vi "Configuration - SWITCH Properties FGV.vi"(8 "error in (no error)":errorcluster, 11 "Parent Ref in":T1 format="%.0x") -> (0 "error out":errorcluster, 3 "Parent Ref out":T1 format="%.0x")   [LabVIEW 2015, in "DMM-SWITCH-ScanList System Explorer.lvlib"]
uses:
  DMM-SWITCH-ScanList System Explorer.lvlib
  <vilib>/NI Veristand/Custom Device API/Custom Device Item Ref.ctl
  <vilib>/NI Veristand/Custom Device API/Custom Device Channel.ctl
  <vilib>/NI Veristand/Custom Device API/Custom Device Channel Type.ctl
  Shared/Constants.vi
  <vilib>/NI Veristand/Custom Device API/Set Item Property (String).vi
  <vilib>/NI Veristand/Custom Device API/Set Item Property (Boolean).vi
  <vilib>/NI Veristand/Custom Device API/Set Item Property (String Array).vi
  <vilib>/NI Veristand/Custom Device API/Custom Device API.lvlib
  Shared/DMM-SWITCH-ScanList Shared.lvlib
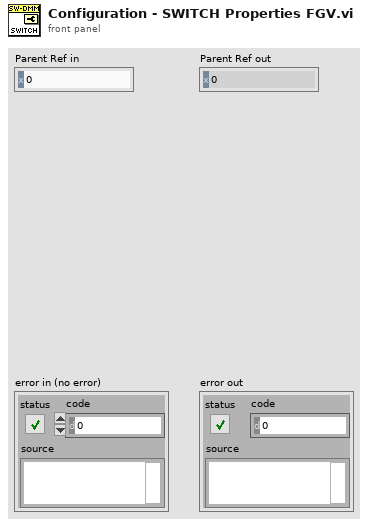
[diagram p1: front panel]
types:
  T1 = typedef "Custom Device API.lvlib/Custom Device Item Ref.ctl" = u64
  T2 = typedef "Custom Device API.lvlib/Custom Device Channel.ctl" = cluster{"Type":T3, "Units":string, "Default Value":dbl, "Faultable":bool, "Scalable":bool}
  T3 = typedef "Custom Device API.lvlib/Custom Device Channel Type.ctl" = enum16{"Input", "Output"}
  T4 = typedef "niSwitch Topologies.ctl" = string
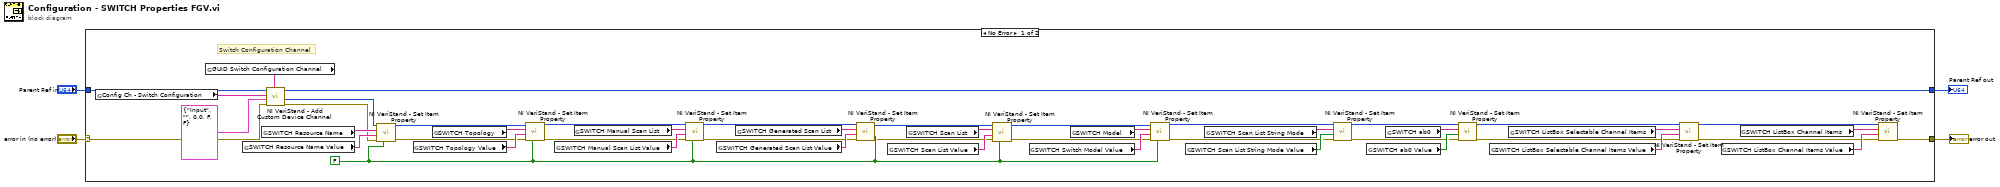
[diagram p0: block diagram]
diagram:
  n1 = case shown="No Error" "error in (no error)" {
    selector: "error in (no error)" -> [w6 w54]
    tunnel: [w18 w54] -> w4
    tunnel: [w9 w53] -> w3
    tunnel: "Parent Ref in" -> [w8 w53]
    frame No Error {
      w30 = FALSE ("Binary String (T)")
      # "Switch Configuration Channel"
      n2 = global read "Constants.vi" "Config Ch - Switch Configuration"() -> (w5:string)
      n3 = global read "Constants.vi" "GUID Switch Configuration Channel"() -> (w40:string)
      n4 = global read "Constants.vi" "SWITCH Resource Name Value"() -> (w31:string)
      n5 = global read "Constants.vi" "SWITCH Resource Name"() -> (w41:string)
      n6 = call <vilib>:"NI VeriStand - Add Custom Device Channel.vi"("GUID (Default Channel)"=w40, "error in (no error)"=w6, "Channel"=T2 {"Type"=enum."Input", "Units"="", "Default Value"=0.0, "Faultable"=FALSE, "Scalable"=FALSE}, "Channel Name"=w5, "Parent Ref in"=w8) -> ("error out"=w13:errorcluster, "Channel Ref"=w12:T1, "Parent Ref out"=w9:T1)  [unwired: 3 in, 1 out]
      n7 = call-poly <vilib>:"NI VeriStand - Set Item Property.vi"("Binary String (T)"=w30, "error in (no error)"=w13, "Value"=w31, "Property Name"=w41, "Item Ref in"=w12) -> ("error out"=w10:errorcluster, "Item Ref out"=w11:T1)  [unwired: 4 in, 1 out]
      n8 = global read "Constants.vi" "SWITCH Topology Value"() -> (w32:T4)
      n9 = global read "Constants.vi" "SWITCH Topology"() -> (w42:string)
      n10 = call-poly <vilib>:"NI VeriStand - Set Item Property.vi"("Binary String (T)"=w30, "error in (no error)"=w10, "Value"=w32, "Property Name"=w42, "Item Ref in"=w11) -> ("error out"=w15:errorcluster, "Item Ref out"=w14:T1)  [unwired: 4 in, 1 out]
      n11 = global read "Constants.vi" "SWITCH Manual Scan List Value"() -> (w33:string)
      n12 = global read "Constants.vi" "SWITCH Manual Scan List"() -> (w43:string)
      n13 = call-poly <vilib>:"NI VeriStand - Set Item Property.vi"("Binary String (T)"=w30, "error in (no error)"=w15, "Value"=w33, "Property Name"=w43, "Item Ref in"=w14) -> ("error out"=w24:errorcluster, "Item Ref out"=w25:T1)  [unwired: 4 in, 1 out]
      n14 = global read "Constants.vi" "SWITCH Generated Scan List Value"() -> (w44:string)
      n15 = global read "Constants.vi" "SWITCH Generated Scan List"() -> (w45:string)
      n16 = call-poly <vilib>:"NI VeriStand - Set Item Property.vi"("Binary String (T)"=w30, "error in (no error)"=w24, "Value"=w44, "Property Name"=w45, "Item Ref in"=w25) -> ("error out"=w28:errorcluster, "Item Ref out"=w26:T1)  [unwired: 4 in, 1 out]
      n17 = global read "Constants.vi" "SWITCH Scan List Value"() -> (w47:string)
      n18 = global read "Constants.vi" "SWITCH Scan List"() -> (w46:string)
      n19 = call-poly <vilib>:"NI VeriStand - Set Item Property.vi"("Binary String (T)"=w30, "error in (no error)"=w28, "Value"=w47, "Property Name"=w46, "Item Ref in"=w26) -> ("error out"=w29:errorcluster, "Item Ref out"=w27:T1)  [unwired: 4 in, 1 out]
      n20 = global read "Constants.vi" "SWITCH Switch Model Value"() -> (w34:string)
      n21 = global read "Constants.vi" "SWITCH Model"() -> (w48:string)
      n22 = call-poly <vilib>:"NI VeriStand - Set Item Property.vi"("Binary String (T)"=w30, "error in (no error)"=w29, "Value"=w34, "Property Name"=w48, "Item Ref in"=w27) -> ("error out"=w20:errorcluster, "Item Ref out"=w19:T1)  [unwired: 4 in, 1 out]
      n23 = global read "Constants.vi" "SWITCH Scan List String Mode Value"() -> (w35:bool)
      n24 = global read "Constants.vi" "SWITCH Scan List String Mode"() -> (w49:string)
      n25 = call-poly <vilib>:"NI VeriStand - Set Item Property.vi"("error in (no error)"=w20, "Value"=w35, "Property Name"=w49, "Item Ref in"=w19) -> ("error out"=w21:errorcluster, "Item Ref out"=w22:T1)  [unwired: 5 in, 1 out]
      n26 = global read "Constants.vi" "SWITCH ab0 Value"() -> (w36:bool)
      n27 = global read "Constants.vi" "SWITCH ab0"() -> (w50:string)
      n28 = call-poly <vilib>:"NI VeriStand - Set Item Property.vi"("error in (no error)"=w21, "Value"=w36, "Property Name"=w50, "Item Ref in"=w22) -> ("error out"=w37:errorcluster, "Item Ref out"=w23:T1)  [unwired: 5 in, 1 out]
      n29 = global read "Constants.vi" "SWITCH ListBox Selectable Channel Items Value"() -> (w38:string[])
      n30 = global read "Constants.vi" "SWITCH ListBox Selectable Channel Items"() -> (w51:string)
      n31 = call-poly <vilib>:"NI VeriStand - Set Item Property.vi"("error in (no error)"=w37, "Value"=w38, "Property Name"=w51, "Item Ref in"=w23) -> ("error out"=w17:errorcluster, "Item Ref out"=w16:T1)  [unwired: 5 in, 1 out]
      n32 = global read "Constants.vi" "SWITCH ListBox Channel Items Value"() -> (w39:string[])
      n33 = global read "Constants.vi" "SWITCH ListBox Channel Items"() -> (w52:string)
      n34 = call-poly <vilib>:"NI VeriStand - Set Item Property.vi"("error in (no error)"=w17, "Value"=w39, "Property Name"=w52, "Item Ref in"=w16) -> ("error out"=w18:errorcluster)  [unwired: 5 in, 2 out]
    }
    frame Error {
    }
  }
  "error out" <- w4
  "Parent Ref out" <- w3
